vi "Make Config File Product.vi"(0 "VISA resource name":refnum<visa-resource-name>, 5 "Command (\"\")":string, 11 "error in (no error)":errorcluster) -> (4 "VISA resource name out":refnum<visa-resource-name>, 6 "Result":string, 15 "error out":errorcluster)   [LabVIEW 2020, in "Yokogawa GX Series.lvlib"]
doc: "Returns result of communication command.\nResult is encoded HEX format."
uses:
  <instrlib>/Yokogawa GX Series/Yokogawa GX Series.lvlib
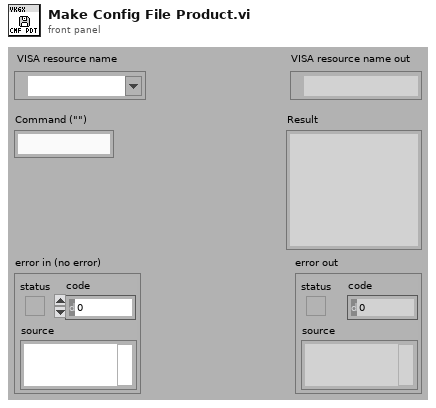
[diagram p1: front panel]
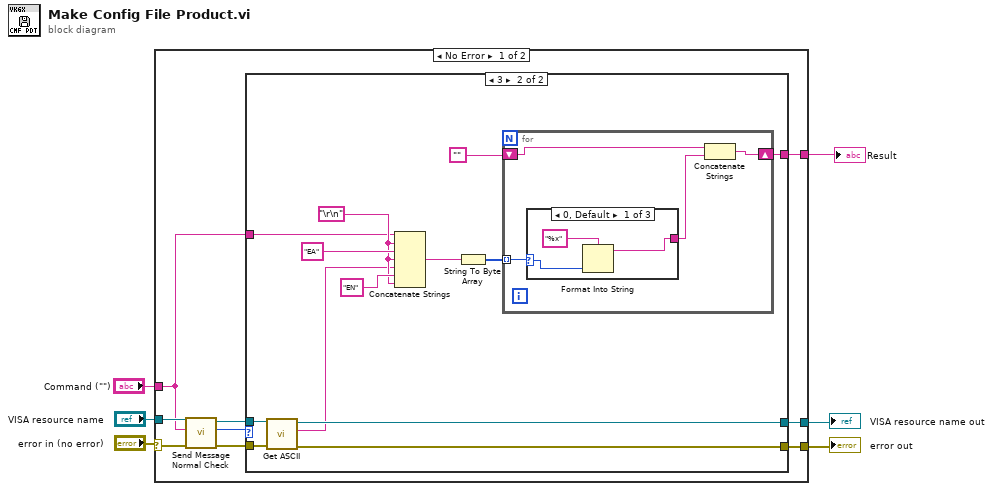
[diagram p0: block diagram]
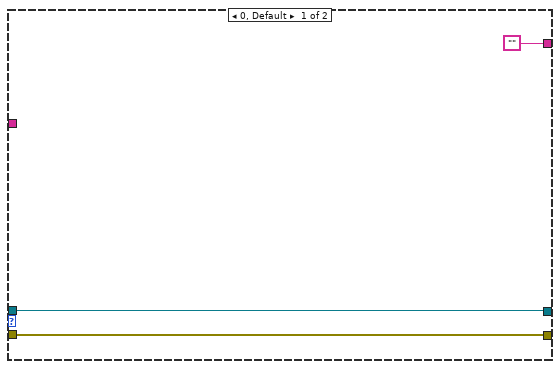
[diagram p2: hidden frame]
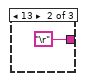
[diagram p3: hidden frame]
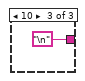
[diagram p4: hidden frame]
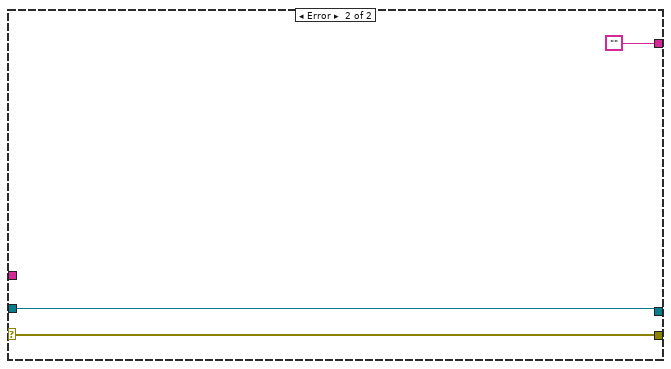
[diagram p5: hidden frame]
diagram:
  n1 = case shown="No Error" "error in (no error)" {
    selector: "error in (no error)" -> [w13 w42]
    tunnel: "Command (\"\")" -> [w7 _]
    tunnel: [w15 ""] -> w5
    tunnel: [w8 w42] -> w3
    tunnel: "VISA resource name" -> [w14 w43]
    tunnel: [w9 w43] -> w1
    frame No Error {
      n2 = call <instrlib>:"Send Message Normal Check.vi"("error in (no error)"=w13, "Send Message (\"\")"=w7, "VISA resource name"=w14) -> ("error out"=w11:errorcluster, "Response Type"=w10:i32, "VISA resource name out"=w12:refnum<visa-resource-name>)  [unwired: 3 in, 3 out]
      n3 = case shown="3" w10 {
        tunnel: ["" w27] -> w15
        tunnel: w12 -> [w17 w24]
        tunnel: w11 -> [w16 w23]
        tunnel: [w17 w22] -> w9
        tunnel: [w16 w21] -> w8
        tunnel: w7 -> [_ w19]
        frame 0, Default {
        }
        frame 3 {
          w25 = "\r\n"
          n4 = call <instrlib>:"Get ASCII.vi"("error in (no error)"=w23, "VISA resource name"=w24) -> ("error out"=w21:errorcluster, "ASCII Data"=w20:string, "VISA resource name out"=w22:refnum<visa-resource-name>)  [unwired: 7 in]
          n5 = Concatenate Strings(w19, w25, "EA", w25, w20, "EN", w25) -> (w30:string)
          n6 = String To Byte Array(string=w30) -> (unsigned byte array=w29:u8[])
          n7 = for {
            tunnel: w29 -> [w35] mode=indexing
            shift-right: [w32] -> w27
            shift-left: "" -> [w33]
            n8 = case shown="0, Default" w35 {
              selector: w35 -> [w38 _ _]
              tunnel: [w36 "\r" "\n"] -> w34
              frame 0, Default {
                n9 = Format Into String(format string="%x", w38) -> (resulting string=w36:string)  [unwired: 2 in, 1 out]
              }
              frame 13 {
              }
              frame 10 {
              }
            }
            n10 = Concatenate Strings(w33, w34) -> (w32:string)
          }
        }
      }
    }
    frame Error {
    }
  }
  "error out" <- w3
  "VISA resource name out" <- w1
  "Result" <- w5
